vi "VCI_INIT_CONFIG.vi"() -> ()   [LabVIEW 2017]
panel:
  out "VCI_INIT_CONFIG":T1={"AccCode"=0, "AccMask"=4294967295, "Reserved"=0, "Filter"=1, "Timing0"=0, "Timing1"=20, "Mode"=0} {"Timing1" format="%x"; "AccMask" format="%x"; "AccCode" format="%x"}
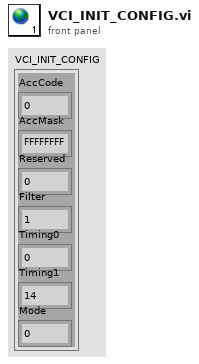
[diagram p1: front panel]
types:
  T1 = cluster{"AccCode":u32, "AccMask":u32, "Reserved":u32, "Filter":u8, "Timing0":u8, "Timing1":u8, "Mode":u8}
diagram:
